vi "Process.vi"(8 "error in":errorcluster, 11 "Edit.Path":refnum<class "Edit.Path.lvclass">) -> (0 "error out":errorcluster, 3 "Edit.Path out":refnum<class "Edit.Path.lvclass">)   [LabVIEW 2019, in "Edit.Path.lvclass"]
doc: "---------------------------------------------------------------\nJKI State Machine Objects™\nhttp://jki.net/state-machine-objects/\nCopyright (C) 2005-2015, JKI <info@jki.net>\nALL RIGHTS RESERVED"
uses:
  Edit.Path.lvclass
  C:/Program Files (x86)/National Instruments/LabVIEW 2019/vi.lib/JKI/JKI SMO/SMO/SMO.lvclass
  <vilib>/JKI/JKI SMO/SMO/Typedefs/Parent Call--Enum.ctl
  Settings/ObjectSettings/ObjectSettings.lvclass/ObjectSettings.ctl
  Settings/Path Settings/Path Settings.lvclass/Path Settings.ctl
  subVIs/typedefs/Schedule Types/Schedule--Constant.ctl
  Settings/Setting Database/Setting Database.lvclass
  Settings/Path Settings/Path Settings.lvclass
  C:/Users/Albro/Documents/GitHub/AFM-Lithography/lvsrc/Classes/Settings/ObjectSettings/ObjectSettings.lvclass
  <vilib>/JKI/JKI SMO/SMO/SMO.lvclass/SMO.ctl
  <vilib>/Utility/miscctls.llb/LVPointTypeDef.ctl
  Settings/Setting Database/Typedefs/PrivateEvents--Setting Database.Copy Settings To Group.ctl
  Settings/Setting Database/Typedefs/PrivateEvents--Setting Database.SetDefaultPath.ctl
  Settings/Setting Database/Typedefs/PrivateEvents--Setting Database.CopyActivePathToAll.ctl
  Settings/ObjectSettings/Accessors/Write Voltage Schedule.vi
  Settings/ObjectSettings/Accessors/Write Speed Schedule.vi
  Settings/ObjectSettings/Accessors/Write Direction.vi
  Settings/ObjectSettings/Accessors/Write Resistance.vi
  Settings/ObjectSettings/Accessors/Write Enabled.vi
  Settings/Path Settings/Accessors/Write Fill Orientation.vi
  Settings/Path Settings/Accessors/Write Smooth Segments.vi
  Settings/ObjectSettings/Accessors/Read Speed Settings.vi
  Settings/ObjectSettings/Accessors/Read Voltage Settings.vi
  Settings/Path Settings/Accessors/Write Fill Spacing.vi
  Settings/Path Settings/Accessors/Write Interpolation.vi
  Settings/Path Settings/Accessors/Read Interpolation.vi
  Settings/ObjectSettings/Accessors/Read Enabled.vi
  Settings/ObjectSettings/Accessors/Read Direction.vi
  Settings/Path Settings/Accessors/Read Fill Orientation.vi
  Settings/Path Settings/Accessors/Read Smooth Segments.vi
  Settings/Path Settings/Accessors/Read Fill Spacing.vi
  Settings/ObjectSettings/Accessors/Read Speed Schedule.vi
  Settings/ObjectSettings/Accessors/Read Voltage Schedule.vi
  Settings/ObjectSettings/Accessors/Read Resistance.vi
  <vilib>/JKI/JKI SMO/SMO/Private/ReftoDVR--SMO.vi
  Edit/Edit.lvclass
  <vilib>/JKI/JKI SMO/SMO/SMO.lvclass
  Settings/ObjectSettings/ObjectSettings.lvclass
panel:
  in  "Apply":bool
  out "Group String":string
  out "ID String":string
  in  "Apply All":bool
  in  "Interpolation":dbl caption="Numeric 2"
  in  "Fill Spacing":dbl caption="Numeric 2"
  in  "Voltage (V)":dbl caption="Numeric 2"
  in  "Speed (um/s)":dbl caption="Numeric 2"
  in  "Smooth Segments":dbl caption="Numeric 2"
  in  "Fill Orientation":u16(ring) caption="Ring" items=["Horizontal", "Vertical"]
  in  "Deviate?":bool=TRUE
  in  "Enabled?":bool=TRUE
  in  "Set Resistance":T1(ring) caption="Enum"
  in  "Direction":u16(ring) caption="Ring" items=["Forward", "Backward"]
  in  "Speed Schedule":u16(ring) caption="Ring" items=["Constant", "Ramp", "Fn. Generator", "Formula"]
  in  "Voltage Schedule":u16(ring) caption="Ring" items=["Constant", "Ramp", "Fn. Generator", "Formula"]
  in  "Speed Settings":bool
  in  "Deviate Settings":bool
  in  "Voltage Settings":bool
  in  "Save Default":bool
  in  "Copy to All":bool
  # "For instructions on how to use the JKI State Machine Objects, examples and video tutorials, visit:\nhttp://jki.net/state-machine-objects/\n\nJKI State Machine Objects™\nhttp://jki.net/state-machine-objects/\nCopyright (C) 2005-2015, JKI <info@jki.net>\nALL RIGHTS RESERVED"
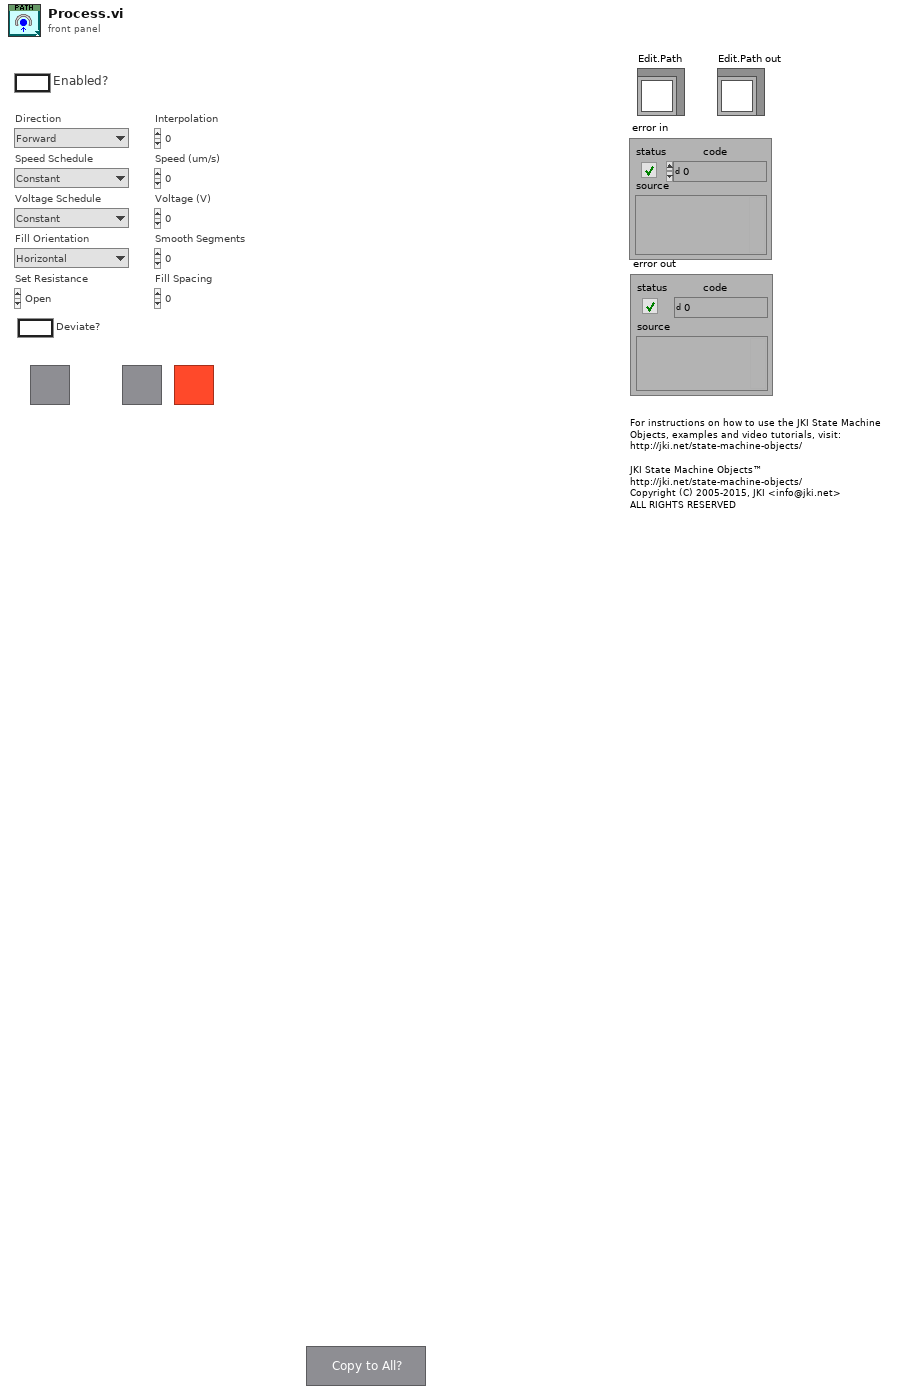
[diagram p1: front panel]
types:
  T1 = enum16{"Open", "Discharge Tip", "0 ohm", "100 kohm", "10 Mohm", "1 Gohm"}
  T2 = typedef "SMO.lvclass/Parent Call--Enum.ctl" = enum16{"Allows parent to run", "Does not request parent to run"}
  T3 = typedef "Schedule--Constant.ctl" = cluster{"Value":dbl}
  T4 = enum32{"invalid app kind", "Development System", "Run Time System", "Student Edition", "Embedded LabVIEW", "Evaluation", "Custom"}
  T5 = typedef "LVPointTypeDef.ctl" = cluster{"Horizontal":i16, "Vertical":i16}
  T6 = enum16{"Always On", "Always Off", "Off While Running"}
  T7 = enum8{"Enabled", "Disabled", "Disabled and Grayed Out"}
  T8 = enum32{"Invalid", "Standard", "Closed", "Hidden", "Minimized", "Maximized"}
  T9 = enum32{"Bad", "Idle", "Run top level", "Running"}
  T10 = typedef "Setting Database.lvclass/PrivateEvents--Setting Database.Copy Settings To Group.ctl" = cluster{"Name":string, "Group":string}
  T11 = typedef "Setting Database.lvclass/PrivateEvents--Setting Database.SetDefaultPath.ctl" = bool
  T12 = typedef "Setting Database.lvclass/PrivateEvents--Setting Database.CopyActivePathToAll.ctl" = bool
  T13 = typedef "Setting Database.lvclass/PublicEvents--Setting Database.NewActivePath.ctl" = refnum<class "Path Settings.lvclass">
  T14 = cluster{"Core":cluster{"Current VI Reference":refnum<vi>, "Close Panel on Exit?":bool, "error":errorcluster}, "Self":refnum<class "Edit.Path.lvclass">, "SettingDB":refnum<class "Setting Database.lvclass">, "Path Settings":refnum<class "Path Settings.lvclass">}
  T15 = cluster{"Current VI Reference":refnum<vi>, "Close Panel on Exit?":bool, "error":errorcluster}
  T16 = typedef "SMO.lvclass/Protected Events.ctl" = cluster{"StopProcesses":refnum<user-event>, "AbortProcesses":refnum<user-event>, "Config Changed":refnum<user-event>, "Dependency":refnum<user-event>}
  T17 = typedef "Setting Database.lvclass/PublicEvents--Cluster.ctl" = cluster{"NewActivePath":refnum<user-event>, "PathsUpdated":refnum<user-event>, "RectanglesUpdated":refnum<user-event>, "NewActiveRectangle":refnum<user-event>, "NewActiveFunnel":refnum<user-event>, "FunnelsUpdated":refnum<user-event>, "NewActiveDot":refnum<user-event>, "DotsUpdated":refnum<user-event>}
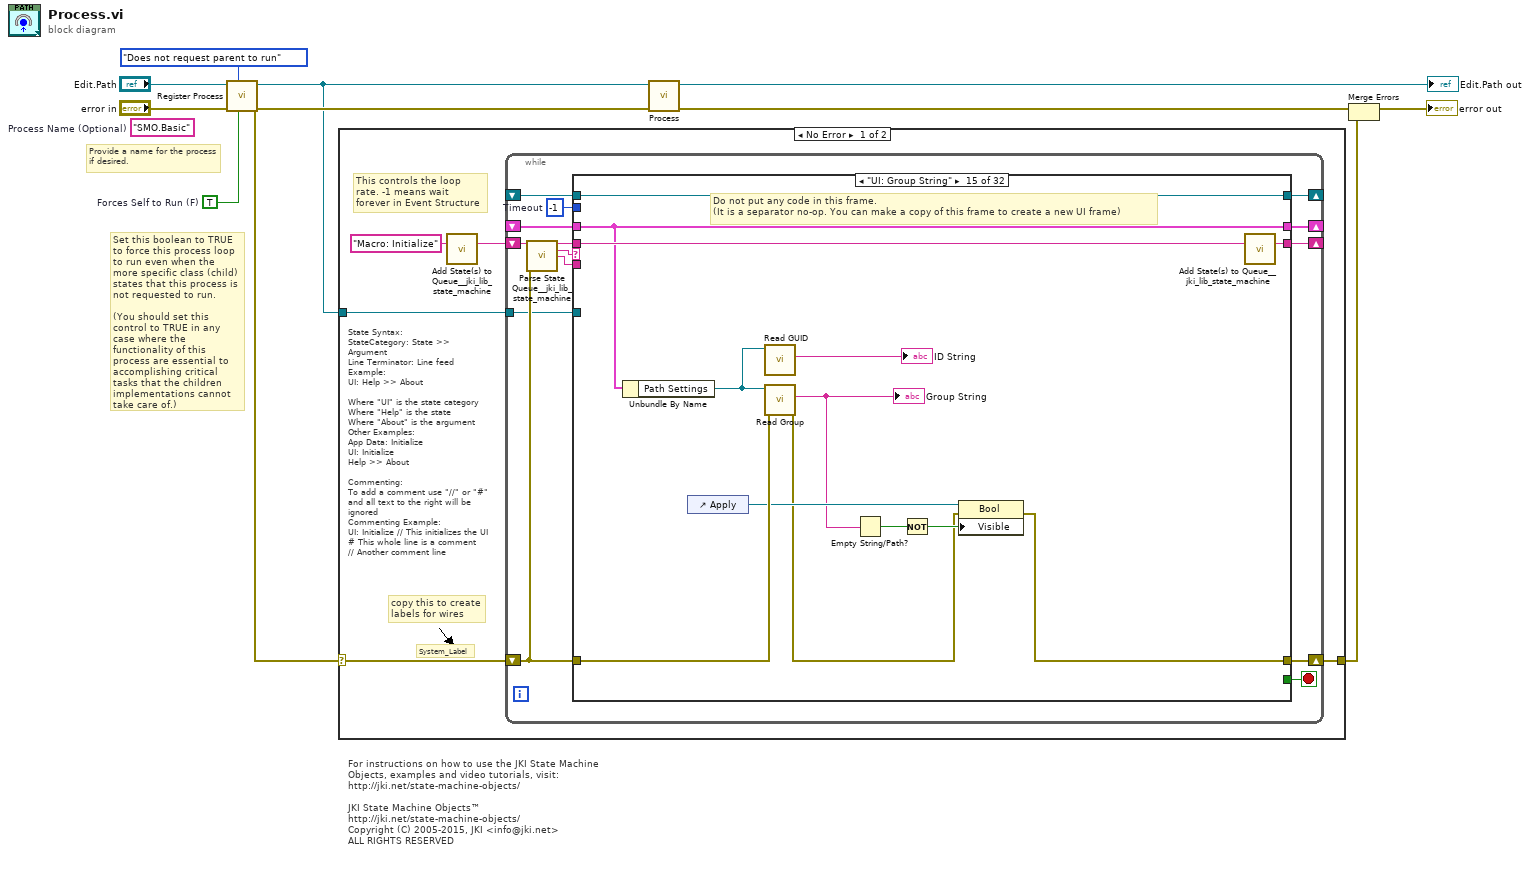
[diagram p0: block diagram]
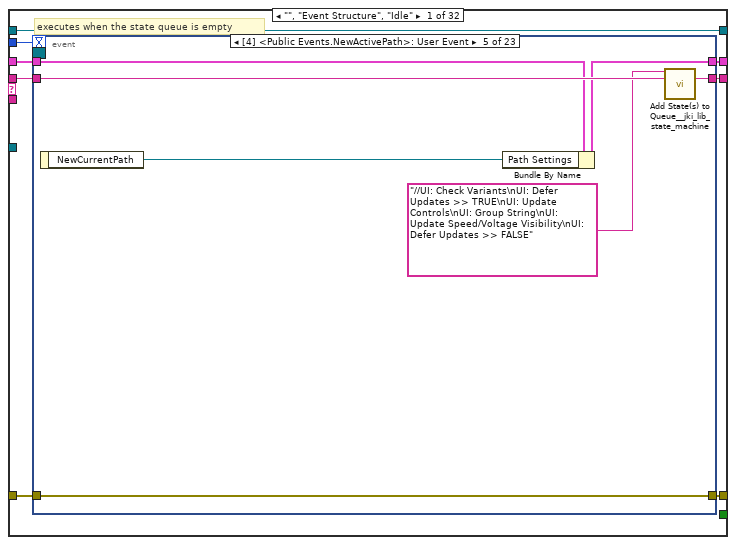
[diagram p2: hidden frame]
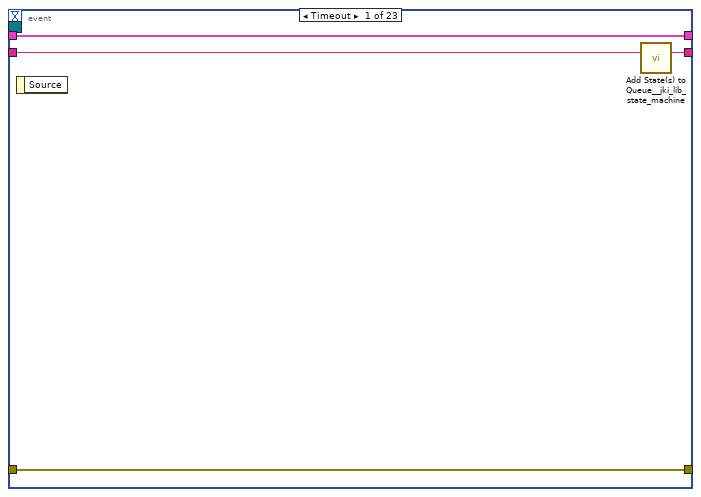
[diagram p3: hidden frame]
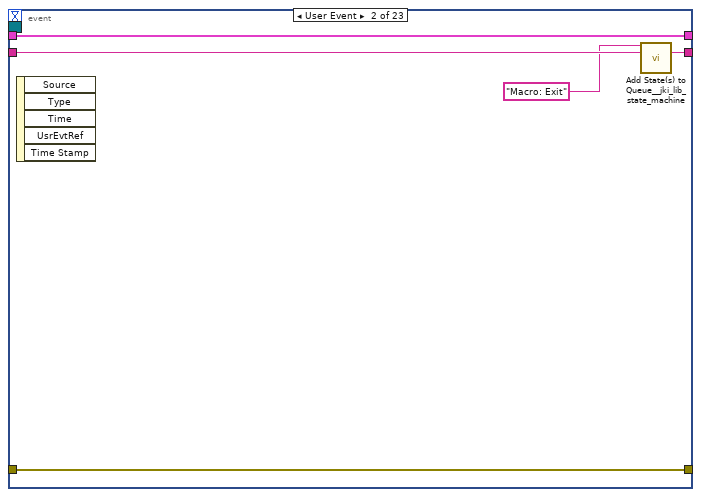
[diagram p4: hidden frame]
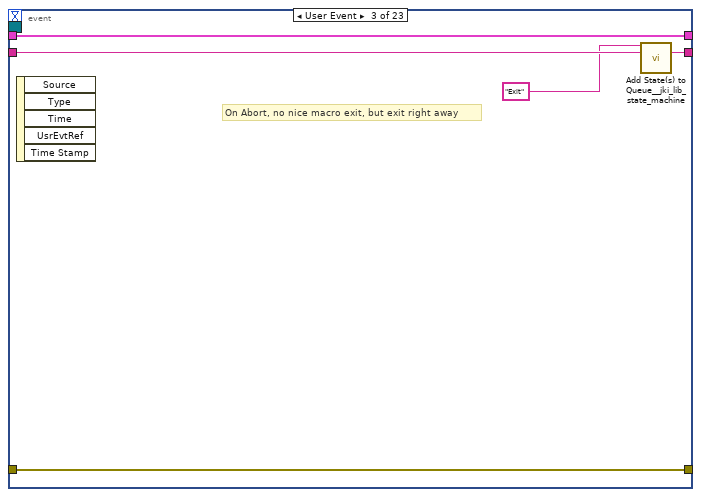
[diagram p5: hidden frame]
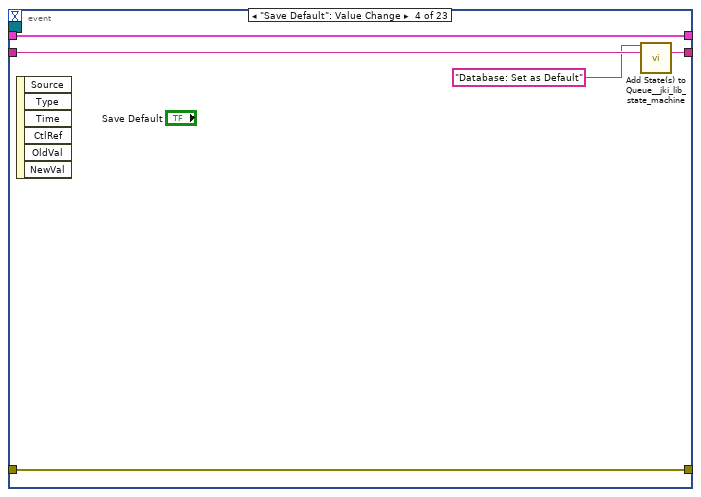
[diagram p6: hidden frame]
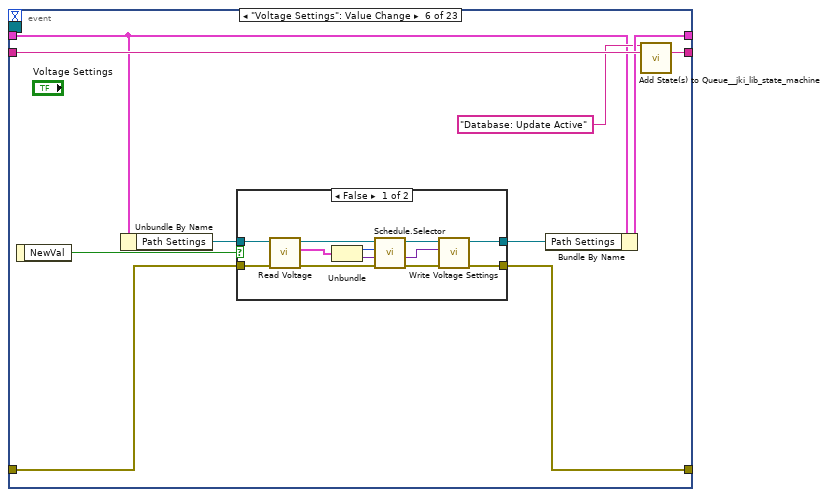
[diagram p7: hidden frame]
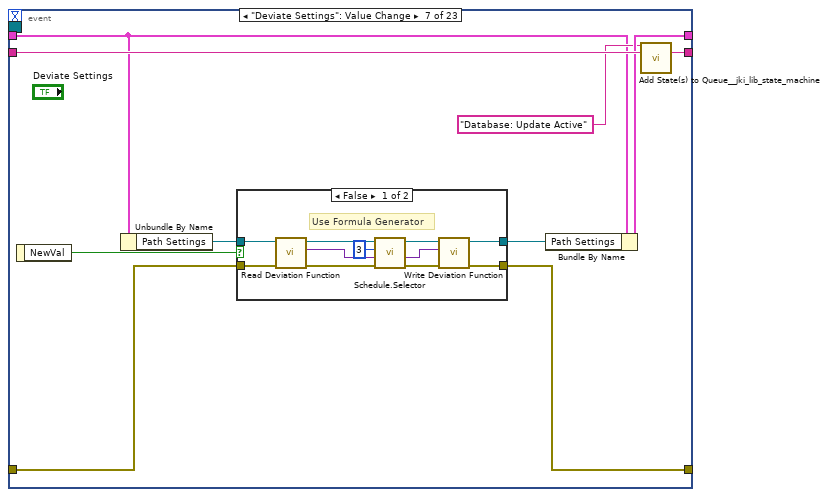
[diagram p9: hidden frame]
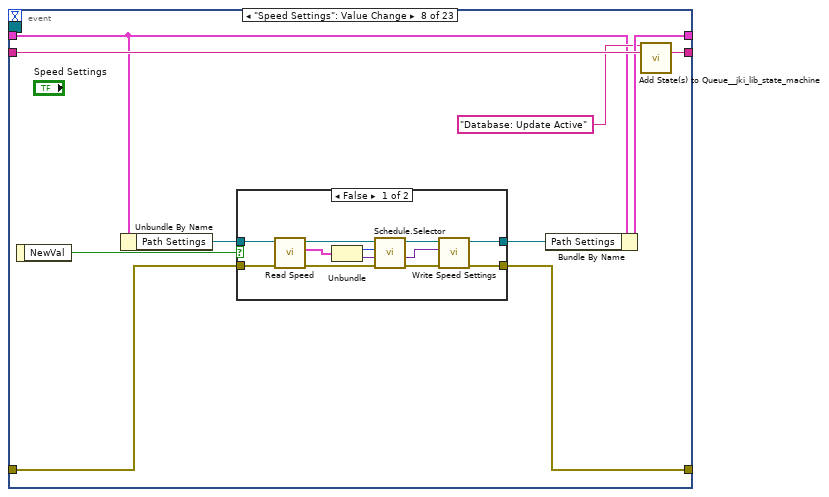
[diagram p11: hidden frame]
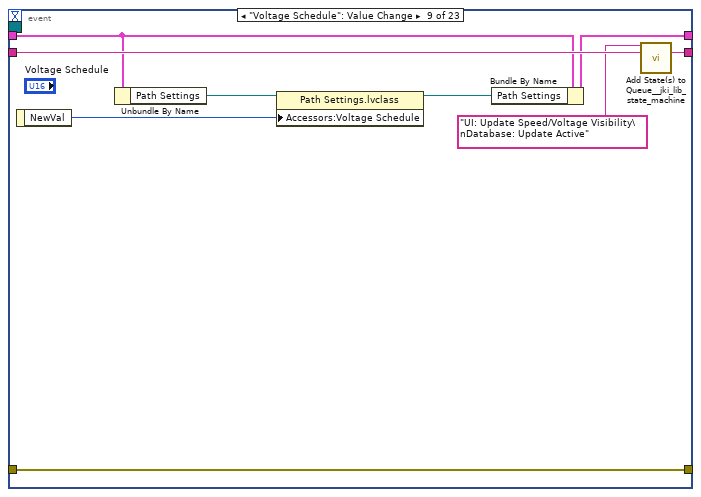
[diagram p13: hidden frame]
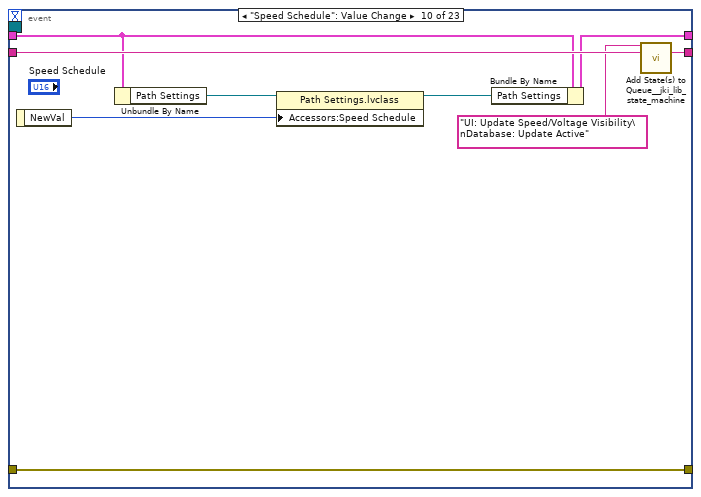
[diagram p14: hidden frame]
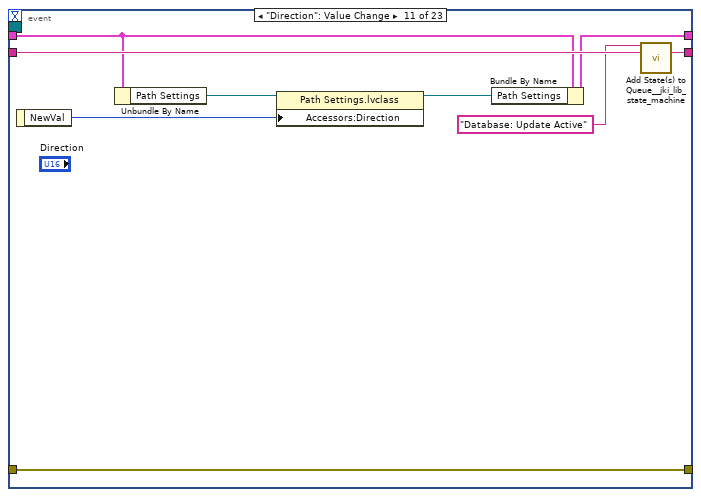
[diagram p15: hidden frame]
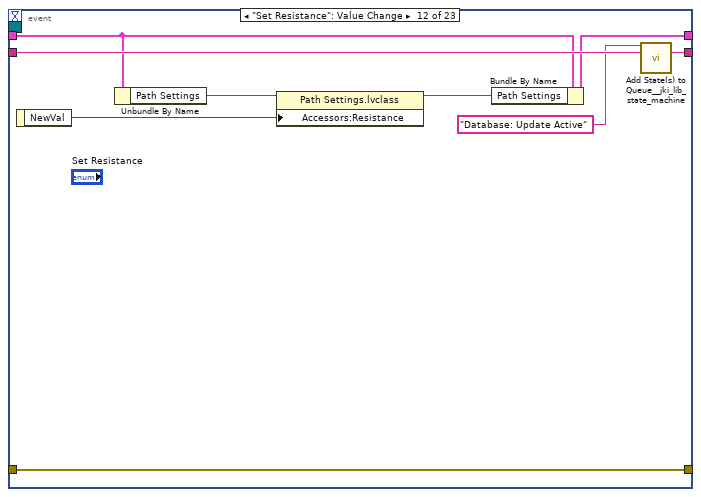
[diagram p16: hidden frame]
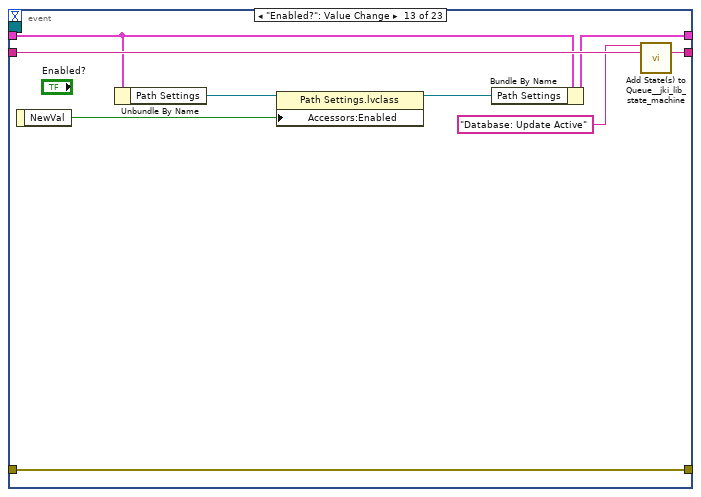
[diagram p17: hidden frame]
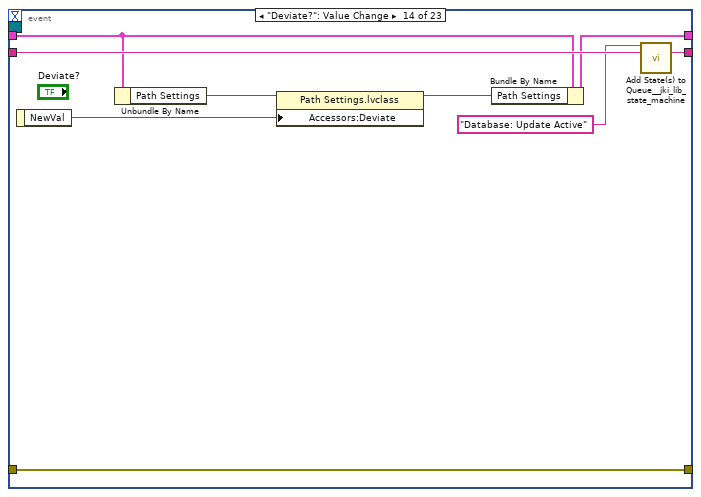
[diagram p18: hidden frame]
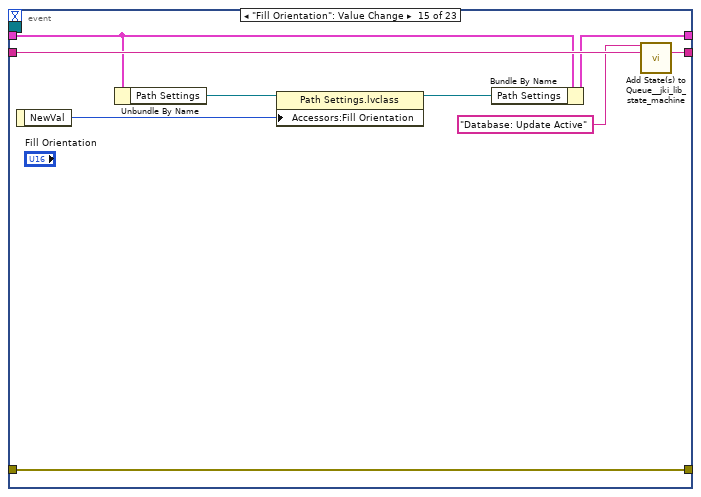
[diagram p19: hidden frame]
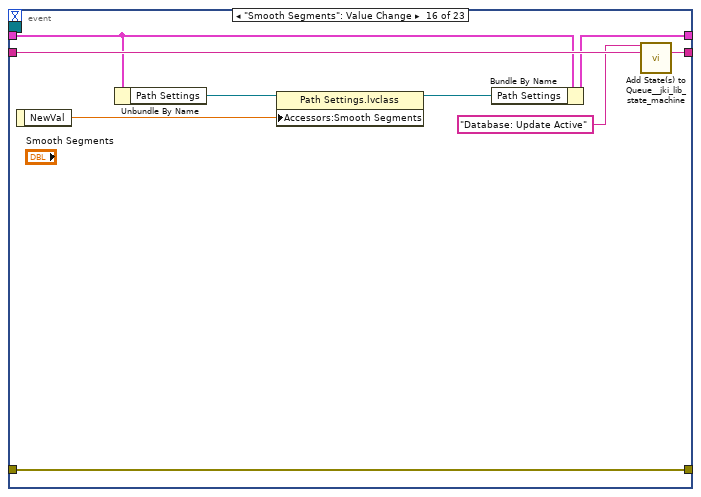
[diagram p20: hidden frame]
diagram:
  w2 = TRUE  # Forces Self to Run (F)
  (unwired) "SMO.Basic"  # Process Name (Optional)
  # "Provide a name for the process\nif desired."
  # "Set this boolean to TRUE to force this process loop to run even when the more specific class (child) states that this process is not requested to run.\n\n(You should set this control to TRUE in any case where the functionality of this process are essential to accomplishing critical tasks that the children implementations cannot take care of.)"
  # "For instructions on how to use the JKI State Machine Objects, examples and video tutorials, visit:\nhttp://jki.net/state-machine-objects/\n\nJKI State Machine Objects™\nhttp://jki.net/state-machine-objects/\nCopyright (C) 2005-2015, JKI <info@jki.net>\nALL RIGHTS RESERVED"
  n1 = call <vilib>:"Register Process.vi"("Forces Self to Run (F)"=w2, "Parent Call"=Parent_Call--Enum."Does not request parent to run", "error in (no error)"="error in", "SMO"="Edit.Path") -> ("error out"=w7:errorcluster, "SMO out"=w1:refnum<class "Edit.Path.lvclass">)  [unwired: 6 in]
  n2 = case shown="No Error" w7 {
    selector: w7 -> [w14 w651]
    tunnel: w1 -> [w13 _]
    tunnel: [w11 w651] -> w4
    frame No Error {
      # "State Syntax:\nStateCategory: State >> Argument\nLine Terminator: Line feed\nExample:\nUI: Help >> About\n\nWhere \"UI\" is the state category\nWhere \"Help\" is the state\nWhere \"About\" is the argument\nOther Examples:\nApp Data: Initialize\nUI: Initialize\nHelp >> About\n\nCommenting:\nTo add a comment use \"//\" or \"#\" and all text to the right will be ignored\nCommenting Example:\nUI: Initialize // This initializes the UI\n# This whole line is a comment\n// Another comment line"
      # "copy this to create labels for wires"
      # "This controls the loop rate. -1 means wait forever in Event Structure"
      # "System_Label"
      n3 = call <vilib>:"Add State(s) to Queue__jki_lib_state_machine.vi"("State(s) in (\"\")"="Macro: Initialize") -> ("States Out"=w12:string)  [unwired: 14 in]
      n4 = while "JKI - String-Based Queued State Machine (Basic) v1.0" {
        shift-right: [w22] -> _
        shift-left: _ -> [w20]
        shift-right: [w25] -> w11
        shift-left: w14 -> [w19]
        shift-right: [w24] -> _
        shift-left: w12 -> [w26]
        shift-right: [w18] -> _
        shift-left: _ -> [w17]
        tunnel: w13 -> [w16]
        stop <- w23 stop-if-true
        w21 = -1  # Timeout
        n5 = call <vilib>:"Parse State Queue__jki_lib_state_machine.vi"("State Queue"=w26, "Error In (no error)"=w19) -> ("Remaining States"=w28:string, "Current State"=w29:string, "Arguments"=w27:string)  [unwired: 11 in]
        n6 = case shown="\"UI: Group String\"" w29 {
          selector: w29 -> [_ _ w281 _ _ _ _ _ _ _ _ _ _ _ _ _ _ _ _ _ _ _ _ _ _ _ _ _ _ _ _ _]
          tunnel: w28 -> [w37 w275 w277 w300 w314 w320 w325 w337 w344 w349 w362 w368 w373 w384 w397 w410 w432 w459 w466 w485 w497 w529 w540 w545 w559 w573 w578 w592 w602 w619 w640 w650]
          tunnel: w27 -> [_ _ _ _ _ _ _ _ _ _ _ _ _ w375 _ _ _ _ w462 _ w493 _ _ _ _ _ _ _ _ _ _ _]
          tunnel: [w34 w273 w284 w298 errorcluster {"status"=FALSE, "code"=0, "source"=""} ("error out") w315 w323 w327 w339 w347 w355 w363 w371 w382 w387 w408 w413 w457 w463 w473 w491 w527 w532 w543 w557 w571 w576 w580 w595 w608 w632 w642] -> w25
          tunnel: w19 -> [w33 w273 w283 w298 w301 _ w323 w326 w340 w347 w353 w364 w371 w382 w393 w408 w416 w457 w464 w481 w492 w527 w531 w543 w557 w571 w576 w579 w594 w605 w631 w641]
          tunnel: [w36 w274 w282 w299 w313 w319 w324 w336 w343 w348 w361 w367 w372 w383 w396 w409 w431 w458 w465 w484 w496 w528 w539 w544 w558 w572 w577 w591 w601 w618 w639 w649] -> w24
          tunnel: [_ _ _ _ _ TRUE _ _ _ _ _ _ _ _ _ _ _ _ _ _ _ _ _ _ _ _ _ _ _ _ _ _] -> w23
          tunnel: [w32 w272 w280 w291 w303 w316 w322 w334 w341 w346 w359 w366 w370 w380 w394 w406 w423 w453 w461 w483 w490 w526 w533 w542 w556 w570 w575 w588 w599 w616 w637 w647] -> w22
          tunnel: w21 -> [w31 _ _ _ _ _ _ _ _ _ _ _ _ _ _ _ _ _ _ _ _ _ _ _ _ _ _ _ _ _ _ _]
          tunnel: w20 -> [w35 w272 w280 w292 w302 w316 w322 _ w341 w346 w359 w366 w370 w380 w394 w405 w423 w453 w461 w483 w490 w526 w533 w542 w556 w570 w575 w587 w598 w604 w636 w646]
          tunnel: [w30 w271 w276 w288 w311 w317 w321 w332 w338 w345 w360 w365 w369 w381 w395 w407 w430 w454 w460 w471 w495 w525 w538 w541 w555 w569 w574 w590 w600 w614 w638 w648] -> w18
          tunnel: w17 -> [w30 w271 w276 w288 w311 w317 w321 w332 w338 w345 _ w365 w369 w381 w395 w407 w430 w454 w460 w471 w495 w525 w538 w541 w555 w569 w574 w590 w600 w614 w638 w648]
          tunnel: w16 -> [_ _ _ _ _ _ _ w330 _ _ _ _ _ _ _ _ _ _ _ _ _ _ _ _ _ _ _ _ _ _ _ _]
          frame "", "Event Structure", "Idle" {
            # "executes when the state queue is empty"
            n7 = event shown="[4] <Public Events.NewActivePath>: User Event" {
              selector: w30 -> [_ _ _ _ _ _ _ _ _ _ _ _ _ _ _ _ _ _ _ _ _ _ _]
              dyn-events: _ -> [_ _ _ _ _ _ _ _ _ _ _ _ _ _ _ _ _ _ _ _ _ _ _]
              timeout: w31 -> [_ _ _ _ _ _ _ _ _ _ _ _ _ _ _ _ _ _ _ _ _ _ _]
              tunnel: w37 -> [w41 w46 w51 w56 w63 w73 w97 w120 w143 w152 w161 w170 w179 w188 w197 w206 w221 w236 w245 w254 w259 w264 w270]
              tunnel: [w40 w45 w50 w55 w62 w72 w96 w119 w142 w151 w160 w169 w178 w187 w196 w205 w220 w235 w244 w253 w258 w263 w269] -> w36
              tunnel: w35 -> [w38 w43 w48 w53 w59 w69 w93 w116 w136 w145 w154 w163 w172 w181 w190 w199 w216 w231 w238 w247 w257 w262 w267]
              tunnel: [w39 w44 w49 w54 w61 w65 w89 w112 w141 w150 w159 w168 w177 w186 w195 w204 w208 w223 w243 w252 w256 w261 w268] -> w34
              tunnel: w33 -> [w39 w44 w49 w54 w61 w64 w88 w111 w141 w150 w159 w168 w177 w186 w195 w204 w207 w222 w243 w252 w256 w261 w268]
              tunnel: [w38 w43 w48 w53 w60 w71 w95 w118 w140 w149 w158 w167 w176 w185 w194 w203 w219 w234 w242 w251 w257 w262 w267] -> w32
              event Timeout {
                n8 = event-data() -> ()  [unwired: 1 in, 1 out]
                n9 = call <vilib>:"Add State(s) to Queue__jki_lib_state_machine.vi"("State(s) in (\"\")"=w41) -> ("States Out"=w40:string)  [unwired: 14 in]
              }
              event User Event {
                n10 = event-data() -> ()  [unwired: 1 in, 5 out]
                n11 = call <vilib>:"Add State(s) to Queue__jki_lib_state_machine.vi"("State(s) in Front (\"\")"="Macro: Exit", "State(s) in (\"\")"=w46) -> ("States Out"=w45:string)  [unwired: 13 in]
              }
              event User Event {
                # "On Abort, no nice macro exit, but exit right away"
                n12 = event-data() -> ()  [unwired: 1 in, 5 out]
                n13 = call <vilib>:"Add State(s) to Queue__jki_lib_state_machine.vi"("State(s) in Front (\"\")"="Exit", "State(s) in (\"\")"=w51) -> ("States Out"=w50:string)  [unwired: 13 in]
              }
              event "Save Default": Value Change {
                n14 = event-data() -> ()  [unwired: 1 in, 6 out]
                n15 = call <vilib>:"Add State(s) to Queue__jki_lib_state_machine.vi"("State(s) in Front (\"\")"="Database: Set as Default", "State(s) in (\"\")"=w56) -> ("States Out"=w55:string)  [unwired: 13 in]
              }
              event User Event {
                n16 = event-data() -> ("NewCurrentPath"=w57:T13)  [unwired: 1 in]
                n17 = Bundle By Name(cluster=w59, "Path Settings"=w57) -> (w60:T14)
                n18 = call <vilib>:"Add State(s) to Queue__jki_lib_state_machine.vi"("State(s) in Front (\"\")"="//UI: Check Variants\nUI: Defer Updates >> TRUE\nUI: Update Controls\nUI: Group String\nUI: Update Speed/Voltage Visibility\nUI: Defer Updates >> FALSE", "State(s) in (\"\")"=w63) -> ("States Out"=w62:string)  [unwired: 13 in]
              }
              event "Voltage Settings": Value Change {
                n19 = event-data() -> ("NewVal"=w68:bool)  [unwired: 1 in]
                n20 = Unbundle By Name(w69) -> ("Path Settings"=w67:refnum<class "Path Settings.lvclass">)
                n21 = case shown="False" w68 {
                  tunnel: w67 -> [w85 w87]
                  tunnel: [w77 w87] -> w66
                  tunnel: w64 -> [w84 w86]
                  tunnel: [w74 w86] -> w65
                  frame False {
                    n22 = call "Read Voltage.vi"("error in (no error)"=w84, "ObjectSettings in"=w85) -> ("error out"=w82:errorcluster, "Voltage"=w81:cluster{"Schedule":u16, "Settings":variant}, "ObjectSettings out"=w83:refnum<class "Path Settings.lvclass">)  [unwired: 7 in]
                    n23 = Unbundle(w81) -> ("Schedule"=w80:u16, "Settings"=w79:variant)
                    n24 = call-dynamic "Schedule.Selector.vi"("error in (no error)"=w82, "Settings In"=w79, "Schedule"=w80, "ObjectSettings in"=w83) -> ("error out"=w76:errorcluster, "Settings Out"=w75:variant, "ObjectSettings out"=w78:refnum<class "Path Settings.lvclass">)  [unwired: 5 in]
                    n25 = call "Write Voltage Settings.vi"("error in (no error)"=w76, "Settings"=w75, "ObjectSettings in"=w78) -> ("error out"=w74:errorcluster, "ObjectSettings out"=w77:refnum<class "Path Settings.lvclass">)  [unwired: 7 in]
                  }
                  frame True {
                  }
                }
                n26 = Bundle By Name(cluster=w69, "Path Settings"=w66) -> (w71:T14)
                n27 = call <vilib>:"Add State(s) to Queue__jki_lib_state_machine.vi"("State(s) in Front (\"\")"="Database: Update Active", "State(s) in (\"\")"=w73) -> ("States Out"=w72:string)  [unwired: 13 in]
              }
              event "Deviate Settings": Value Change {
                n28 = event-data() -> ("NewVal"=w92:bool)  [unwired: 1 in]
                n29 = Unbundle By Name(w93) -> ("Path Settings"=w91:refnum<class "Path Settings.lvclass">)
                n30 = case shown="False" w92 {
                  tunnel: w91 -> [w103 w110]
                  tunnel: [w107 w110] -> w90
                  tunnel: w88 -> [w100 w109]
                  tunnel: [w104 w109] -> w89
                  frame False {
                    # "Use Formula Generator"
                    n31 = call-dynamic "Read Deviation Function.vi"("error in (no error)"=w100, "Path Settings in"=w103) -> ("error out"=w101:errorcluster, "Deviation Function"=w99:variant, "Path Settings out"=w102:refnum<class "Path Settings.lvclass">)  [unwired: 7 in]
                    n32 = call-dynamic "Schedule.Selector.vi"("error in (no error)"=w101, "Settings In"=w99, "Schedule"=u16 3, "ObjectSettings in"=w102) -> ("error out"=w106:errorcluster, "Settings Out"=w105:variant, "ObjectSettings out"=w108:refnum<class "Path Settings.lvclass">)  [unwired: 5 in]
                    n33 = call-dynamic "Write Deviation Function.vi"("error in (no error)"=w106, "Deviation Function"=w105, "Path Settings in"=w108) -> ("error out"=w104:errorcluster, "Path Settings out"=w107:refnum<class "Path Settings.lvclass">)  [unwired: 7 in]
                  }
                  frame True {
                  }
                }
                n34 = Bundle By Name(cluster=w93, "Path Settings"=w90) -> (w95:T14)
                n35 = call <vilib>:"Add State(s) to Queue__jki_lib_state_machine.vi"("State(s) in Front (\"\")"="Database: Update Active", "State(s) in (\"\")"=w97) -> ("States Out"=w96:string)  [unwired: 13 in]
              }
              event "Speed Settings": Value Change {
                n36 = event-data() -> ("NewVal"=w115:bool)  [unwired: 1 in]
                n37 = Unbundle By Name(w116) -> ("Path Settings"=w114:refnum<class "Path Settings.lvclass">)
                n38 = case shown="False" w115 {
                  tunnel: w114 -> [w130 w134]
                  tunnel: [w124 w134] -> w113
                  tunnel: w111 -> [w128 w133]
                  tunnel: [w123 w133] -> w112
                  frame False {
                    n39 = call "Read Speed.vi"("error in (no error)"=w128, "ObjectSettings in"=w130) -> ("error out"=w127:errorcluster, "Speed"=w126:cluster{"Schedule":u16, "Settings":variant}, "ObjectSettings out"=w129:refnum<class "Path Settings.lvclass">)  [unwired: 7 in]
                    n40 = Unbundle(w126) -> ("Schedule"=w132:u16, "Settings"=w131:variant)
                    n41 = call-dynamic "Schedule.Selector.vi"("error in (no error)"=w127, "Settings In"=w131, "Schedule"=w132, "ObjectSettings in"=w129) -> ("error out"=w122:errorcluster, "Settings Out"=w121:variant, "ObjectSettings out"=w125:refnum<class "Path Settings.lvclass">)  [unwired: 5 in]
                    n42 = call "Write Speed Settings.vi"("error in (no error)"=w122, "Settings"=w121, "ObjectSettings in"=w125) -> ("error out"=w123:errorcluster, "ObjectSettings out"=w124:refnum<class "Path Settings.lvclass">)  [unwired: 7 in]
                  }
                  frame True {
                  }
                }
                n43 = Bundle By Name(cluster=w116, "Path Settings"=w113) -> (w118:T14)
                n44 = call <vilib>:"Add State(s) to Queue__jki_lib_state_machine.vi"("State(s) in Front (\"\")"="Database: Update Active", "State(s) in (\"\")"=w120) -> ("States Out"=w119:string)  [unwired: 13 in]
              }
              event "Voltage Schedule": Value Change {
                n45 = event-data() -> ("NewVal"=w135:u16)  [unwired: 1 in]
                n46 = Unbundle By Name(w136) -> ("Path Settings"=w138:refnum<class "Path Settings.lvclass">)
                n47 = property class="Path Settings.lvclass"(reference=w138, "Accessors:Voltage Schedule"=w135) -> (reference out=w137:refnum<class "Path Settings.lvclass">)  [unwired: 1 in, 1 out]
                n48 = Bundle By Name(cluster=w136, "Path Settings"=w137) -> (w140:T14)
                n49 = call <vilib>:"Add State(s) to Queue__jki_lib_state_machine.vi"("State(s) in Front (\"\")"="UI: Update Speed/Voltage Visibility\nDatabase: Update Active", "State(s) in (\"\")"=w143) -> ("States Out"=w142:string)  [unwired: 13 in]
              }
              event "Speed Schedule": Value Change {
                n50 = event-data() -> ("NewVal"=w144:u16)  [unwired: 1 in]
                n51 = Unbundle By Name(w145) -> ("Path Settings"=w147:refnum<class "Path Settings.lvclass">)
                n52 = property class="Path Settings.lvclass"(reference=w147, "Accessors:Speed Schedule"=w144) -> (reference out=w146:refnum<class "Path Settings.lvclass">)  [unwired: 1 in, 1 out]
                n53 = Bundle By Name(cluster=w145, "Path Settings"=w146) -> (w149:T14)
                n54 = call <vilib>:"Add State(s) to Queue__jki_lib_state_machine.vi"("State(s) in Front (\"\")"="UI: Update Speed/Voltage Visibility\nDatabase: Update Active", "State(s) in (\"\")"=w152) -> ("States Out"=w151:string)  [unwired: 13 in]
              }
              event "Direction": Value Change {
                n55 = event-data() -> ("NewVal"=w153:u16)  [unwired: 1 in]
                n56 = Unbundle By Name(w154) -> ("Path Settings"=w156:refnum<class "Path Settings.lvclass">)
                n57 = property class="Path Settings.lvclass"(reference=w156, "Accessors:Direction"=w153) -> (reference out=w155:refnum<class "Path Settings.lvclass">)  [unwired: 1 in, 1 out]
                n58 = Bundle By Name(cluster=w154, "Path Settings"=w155) -> (w158:T14)
                n59 = call <vilib>:"Add State(s) to Queue__jki_lib_state_machine.vi"("State(s) in Front (\"\")"="Database: Update Active", "State(s) in (\"\")"=w161) -> ("States Out"=w160:string)  [unwired: 13 in]
              }
              event "Set Resistance": Value Change {
                n60 = event-data() -> ("NewVal"=w162:T1)  [unwired: 1 in]
                n61 = Unbundle By Name(w163) -> ("Path Settings"=w165:refnum<class "Path Settings.lvclass">)
                n62 = property class="Path Settings.lvclass"(reference=w165, "Accessors:Resistance"=w162) -> (reference out=w164:refnum<class "Path Settings.lvclass">)  [unwired: 1 in, 1 out]
                n63 = Bundle By Name(cluster=w163, "Path Settings"=w164) -> (w167:T14)
                n64 = call <vilib>:"Add State(s) to Queue__jki_lib_state_machine.vi"("State(s) in Front (\"\")"="Database: Update Active", "State(s) in (\"\")"=w170) -> ("States Out"=w169:string)  [unwired: 13 in]
              }
              event "Enabled?": Value Change {
                n65 = event-data() -> ("NewVal"=w171:bool)  [unwired: 1 in]
                n66 = Unbundle By Name(w172) -> ("Path Settings"=w174:refnum<class "Path Settings.lvclass">)
                n67 = property class="Path Settings.lvclass"(reference=w174, "Accessors:Enabled"=w171) -> (reference out=w173:refnum<class "Path Settings.lvclass">)  [unwired: 1 in, 1 out]
                n68 = Bundle By Name(cluster=w172, "Path Settings"=w173) -> (w176:T14)
                n69 = call <vilib>:"Add State(s) to Queue__jki_lib_state_machine.vi"("State(s) in Front (\"\")"="Database: Update Active", "State(s) in (\"\")"=w179) -> ("States Out"=w178:string)  [unwired: 13 in]
              }
              event "Deviate?": Value Change {
                n70 = event-data() -> ("NewVal"=w180:bool)  [unwired: 1 in]
                n71 = Unbundle By Name(w181) -> ("Path Settings"=w183:refnum<class "Path Settings.lvclass">)
                n72 = property class="Path Settings.lvclass"(reference=w183, "Accessors:Deviate"=w180) -> (reference out=w182:refnum<class "Path Settings.lvclass">)  [unwired: 1 in, 1 out]
                n73 = Bundle By Name(cluster=w181, "Path Settings"=w182) -> (w185:T14)
                n74 = call <vilib>:"Add State(s) to Queue__jki_lib_state_machine.vi"("State(s) in Front (\"\")"="Database: Update Active", "State(s) in (\"\")"=w188) -> ("States Out"=w187:string)  [unwired: 13 in]
              }
              event "Fill Orientation": Value Change {
                n75 = event-data() -> ("NewVal"=w189:u16)  [unwired: 1 in]
                n76 = Unbundle By Name(w190) -> ("Path Settings"=w192:refnum<class "Path Settings.lvclass">)
                n77 = property class="Path Settings.lvclass"(reference=w192, "Accessors:Fill Orientation"=w189) -> (reference out=w191:refnum<class "Path Settings.lvclass">)  [unwired: 1 in, 1 out]
                n78 = Bundle By Name(cluster=w190, "Path Settings"=w191) -> (w194:T14)
                n79 = call <vilib>:"Add State(s) to Queue__jki_lib_state_machine.vi"("State(s) in Front (\"\")"="Database: Update Active", "State(s) in (\"\")"=w197) -> ("States Out"=w196:string)  [unwired: 13 in]
              }
              event "Smooth Segments": Value Change {
                n80 = event-data() -> ("NewVal"=w198:dbl)  [unwired: 1 in]
                n81 = Unbundle By Name(w199) -> ("Path Settings"=w201:refnum<class "Path Settings.lvclass">)
                n82 = property class="Path Settings.lvclass"(reference=w201, "Accessors:Smooth Segments"=w198) -> (reference out=w200:refnum<class "Path Settings.lvclass">)  [unwired: 1 in, 1 out]
                n83 = Bundle By Name(cluster=w199, "Path Settings"=w200) -> (w203:T14)
                n84 = call <vilib>:"Add State(s) to Queue__jki_lib_state_machine.vi"("State(s) in Front (\"\")"="Database: Update Active", "State(s) in (\"\")"=w206) -> ("States Out"=w205:string)  [unwired: 13 in]
              }
              event "Speed (um/s)": Value Change {
                n85 = event-data() -> ("NewVal"=w214:dbl)  [unwired: 1 in]
                n86 = Unbundle By Name(w216) -> ("Path Settings"=w213:refnum<class "Path Settings.lvclass">)
                n87 = property class="Path Settings.lvclass"(reference=w213) -> (reference out=w212:refnum<class "Path Settings.lvclass">, "Accessors:Speed Settings"=w211:variant)  [unwired: 1 in, 1 out]
                n88 = Bundle By Name(cluster=T3 {"Value"=10.0} ("Constant"), "Value"=w214) -> (w209:T3)
                n89 = call "Schedule.Write.vi"("error in (no error)"=w207, "Data to Write"=w209, "LUT In"=w211) -> ("error out"=w208:errorcluster, "LUT Out"=w210:variant)  [unwired: 7 in]
                n90 = property class="Path Settings.lvclass"(reference=w212, "Accessors:Speed Settings"=w210) -> (reference out=w217:refnum<class "Path Settings.lvclass">)  [unwired: 1 in, 1 out]
                n91 = Bundle By Name(cluster=w216, "Path Settings"=w217) -> (w219:T14)
                n92 = call <vilib>:"Add State(s) to Queue__jki_lib_state_machine.vi"("State(s) in Front (\"\")"="Database: Update Active", "State(s) in (\"\")"=w221) -> ("States Out"=w220:string)  [unwired: 13 in]
              }
              event "Voltage (V)": Value Change {
                n93 = event-data() -> ("NewVal"=w229:dbl)  [unwired: 1 in]
                n94 = Unbundle By Name(w231) -> ("Path Settings"=w228:refnum<class "Path Settings.lvclass">)
                n95 = property class="Path Settings.lvclass"(reference=w228) -> (reference out=w227:refnum<class "Path Settings.lvclass">, "Accessors:Voltage Settings"=w226:variant)  [unwired: 1 in, 1 out]
                n96 = Bundle By Name(cluster=T3 {"Value"=10.0} ("Constant"), "Value"=w229) -> (w224:T3)
                n97 = call "Schedule.Write.vi"("error in (no error)"=w222, "Data to Write"=w224, "LUT In"=w226) -> ("error out"=w223:errorcluster, "LUT Out"=w225:variant)  [unwired: 7 in]
                n98 = property class="Path Settings.lvclass"(reference=w227, "Accessors:Voltage Settings"=w225) -> (reference out=w232:refnum<class "Path Settings.lvclass">)  [unwired: 1 in, 1 out]
                n99 = Bundle By Name(cluster=w231, "Path Settings"=w232) -> (w234:T14)
                n100 = call <vilib>:"Add State(s) to Queue__jki_lib_state_machine.vi"("State(s) in Front (\"\")"="Database: Update Active", "State(s) in (\"\")"=w236) -> ("States Out"=w235:string)  [unwired: 13 in]
              }
              event "Fill Spacing": Value Change {
                n101 = event-data() -> ("NewVal"=w237:dbl)  [unwired: 1 in]
                n102 = Unbundle By Name(w238) -> ("Path Settings"=w240:refnum<class "Path Settings.lvclass">)
                n103 = property class="Path Settings.lvclass"(reference=w240, "Accessors:Fill Spacing"=w237) -> (reference out=w239:refnum<class "Path Settings.lvclass">)  [unwired: 1 in, 1 out]
                n104 = Bundle By Name(cluster=w238, "Path Settings"=w239) -> (w242:T14)
                n105 = call <vilib>:"Add State(s) to Queue__jki_lib_state_machine.vi"("State(s) in Front (\"\")"="Database: Update Active", "State(s) in (\"\")"=w245) -> ("States Out"=w244:string)  [unwired: 13 in]
              }
              event "Interpolation": Value Change {
                n106 = event-data() -> ("NewVal"=w246:dbl)  [unwired: 1 in]
                n107 = Unbundle By Name(w247) -> ("Path Settings"=w249:refnum<class "Path Settings.lvclass">)
                n108 = property class="Path Settings.lvclass"(reference=w249, "Accessors:Interpolation"=w246) -> (reference out=w248:refnum<class "Path Settings.lvclass">)  [unwired: 1 in, 1 out]
                n109 = Bundle By Name(cluster=w247, "Path Settings"=w248) -> (w251:T14)
                n110 = call <vilib>:"Add State(s) to Queue__jki_lib_state_machine.vi"("State(s) in Front (\"\")"="Database: Update Active", "State(s) in (\"\")"=w254) -> ("States Out"=w253:string)  [unwired: 13 in]
              }
              event "Copy to All", "Apply All": Value Change {
                n111 = event-data() -> ()  [unwired: 1 in, 1 out]
                n112 = call <vilib>:"Add State(s) to Queue__jki_lib_state_machine.vi"("State(s) in Front (\"\")"="Database: Copy to All", "State(s) in (\"\")"=w259) -> ("States Out"=w258:string)  [unwired: 13 in]
              }
              event "Apply": Value Change {
                n113 = event-data() -> ()  [unwired: 1 in, 1 out]
                n114 = call <vilib>:"Add State(s) to Queue__jki_lib_state_machine.vi"("State(s) in Front (\"\")"="Database: Copy to Group", "State(s) in (\"\")"=w264) -> ("States Out"=w263:string)  [unwired: 13 in]
              }
              event Panel Close? {
                # "Discard the event because we'll close the front panel ourselves in Macro: Exit"
                # "Close Panel button (pressed) Event\n(this executes Macro: Exit to terminate the VI)"
                n115 = event-data() -> ()  [unwired: 1 in, 1 out]
                n116 = event-data("Discard?"=TRUE) -> ()  [unwired: 1 in, 1 out]
                n117 = call <vilib>:"Add State(s) to Queue__jki_lib_state_machine.vi"("State(s) in Front (\"\")"="Macro: Exit", "State(s) in (\"\")"=w270) -> ("States Out"=w269:string)  [unwired: 13 in]
              }
            }
          }
          frame "---------- Core ----------" {
            # "Do not put any code in this frame.\n(it is a separator no-op)"
            n118 = call <vilib>:"Add State(s) to Queue__jki_lib_state_machine.vi"("State(s) in (\"\")"=w275) -> ("States Out"=w274:string)  [unwired: 14 in]
          }
          frame Default {
            w287 = 42 items=["No error", "Argument error", "Memory is full", "Out of zone", "End of file", "File already open", "Generic file I/O error", "File not found", "File permission error", "Disk is full", "Duplicate path", "Too many files open", "System feature not enabled", "Resource file not found", "Cannot add resource", "Resource not found", "Image not found", "Image memory error", "Pen does not exist", "Config type invalid", "Config token not found", "Config parse error", "Config memory error", "Bad external code format", "Bad external code offset", "External code not present", "Null window", "Destroy window error", "Null menu", "Print aborted", "Bad print record", "Print driver error", "Windows error during printing", "Memory error during printing", "Print dialog error", "Generic print error", "Invalid device refnum", "Device not found", "Device parameter error", "Device unit error", "Cannot open device", "Device call aborted", "Generic error", "Cancelled by user", "Object ID too low", "Object ID too high", "Object not in heap", "Unknown heap", "Unknown object (invalid DefProc)", "Unknown object (DefProc not in table)", "Message out of range", "Invalid (null) method", "Unknown message", "Manager call not supported", "Bad address", "Network operation in progress", "Network operation timed out", "Connection is busy", "Network attribute not supported", "Network error", "Address in use", "System out of memory", "Connection aborted", "Connection refused", "Not connected", "Already connected", "Connection closed", "Initialization error (interapplication manager)", "Bad occurrence", "Wait on unbound occurrence handler", "Occurrence queue overflow", "Datalog type conflict", "Unused", "Unrecognized type (interapplication manager)", "Memory corrupt", "Failed to make temporary DLL", "Old CIN version", "Drag socket not found", "Failed to load drop-object", "Failed to register OLE object", "Failed to release OLE object", "Format specifier type mismatch", "Unknown format specifier", "Too few format specifiers", "Too many format specifiers", "Scan failed", "Newer CIN version", "Error converting to variant", "Runtime menu error", "Password tampered", "Variant attribute not found", "Incompatible variant data type", "Event data is not available", "Event Store is not present", "Occurrence is not found", "Event Queue is not created", "Event info is not available", "Refnum passed is NULL", "Error retrieving Class GUID", "Error retrieving CoClass GUID", "Error retrieving TypeLib GUID.", "Bad built application magic bytes.", "Specific driver is different from the specific driver associated with the Logical Name.", "There is no session opened to the class driver.", "Max Error", "MAX - Error with config objects", "MAX - Error loading configuration", "MAX - Group not supported"]
            # "Current State"
            # "Do not delete, rename, or modify this frame.\n(this is used to capture unhandled states and typos)"
            # "Handle mistyped state name (developer tool)"
            n119 = Format Into String(format string="Software Exception: Unhandled State \"%s\"." ("message"), error in=w283, w281) -> (resulting string=w286:string, error out=w285:errorcluster)  [unwired: 1 in]
            n120 = call <vilib>:"Error Cluster From Error Code.vi"("show call chain? (False)"=TRUE, "error in (no error)"=w285, "error message (\"\")"=w286, "error code (0)"=w287) -> ("error out"=w284:errorcluster)  [unwired: 5 in]
            n121 = call <vilib>:"Add State(s) to Queue__jki_lib_state_machine.vi"("State(s) in (\"\")"=w277) -> ("States Out"=w282:string)  [unwired: 14 in]
          }
          frame "Initialize Core Data" {
            # "exe?"
            # "If panel starts closed or is an EXE, then close it when we exit"
            # "Do not delete, rename, or modify this frame.\n(this is used to determine panel behavior on exit)"
            n122 = control-ref of="Current VI Reference"() -> (w297:refnum<vi>)
            n123 = property class="VI"() -> ("Front Panel.Open"=w296:bool)  [unwired: 2 in, 2 out]
            n124 = property class="App"() -> ("App.Kind"=w295:T4)  [unwired: 2 in, 2 out]
            n125 = Not(x=w296) -> (.not. x?=w290:bool)
            n126 = Equal?(x=w295, y=T4."Run Time System" ("Application:Kind")) -> (x = y?=w289:bool)
            n127 = Or(x=w290, y=w289) -> (x .or. y?=w293:bool)
            n128 = Bundle By Name(cluster=w292, "Core.Current VI Reference"=w297, "Core.Close Panel on Exit?"=w293) -> (w291:T14)
            n129 = call <vilib>:"Add State(s) to Queue__jki_lib_state_machine.vi"("State(s) in (\"\")"=w300) -> ("States Out"=w299:string)  [unwired: 14 in]
          }
          frame "Error Handler" {
            w305 = TRUE  # Stop on Unhandled Error (T)
            # "Overwrite this method to handle errors and pass to parent if not handled. Parent will fire a public event if the error is not handled up the chain of classes."
            # "Handle any errors here.\nYou can also output any states to clean-up after errors occur"
            # "Clear error"
            n130 = Unbundle By Name(w302) -> ("Self"=w310:refnum<class "Edit.Path.lvclass">)
            n131 = call-dynamic "Handle Error.vi"("Stop on Unhandled Error (T)"=w305, "error in"=w301, "SMO"=w310) -> ("handling error"=w306:errorcluster, "Unhandled error"=w309:errorcluster)  [unwired: 6 in, 1 out]
            n132 = Bundle By Name(cluster=w302, "Core.error"=w309) -> (w303:T14)
            n133 = Select(t="Exit", s=w306, f="") -> (s? t:f=w304:string)
            n134 = call <vilib>:"Add State(s) to Queue__jki_lib_state_machine.vi"("State(s) in Front (\"\")"=w304, "State(s) in (\"\")"=w314) -> ("States Out"=w313:string)  [unwired: 13 in]
          }
          frame "Exit" {
            # "Do not put any code in this frame.\n(No errors that occur here will be handled.)"
            n135 = Unbundle By Name(w316) -> ("Core.error"=w315:errorcluster)
            n136 = call <vilib>:"Add State(s) to Queue__jki_lib_state_machine.vi"("State(s) in (\"\")"=w320) -> ("States Out"=w319:string)  [unwired: 14 in]
          }
          frame "---------- Data ----------" {
            # "Do not put any code in this frame.\n(It is a separator no-op. You can make a copy of this frame to create a new Data frame)"
            n137 = call <vilib>:"Add State(s) to Queue__jki_lib_state_machine.vi"("State(s) in (\"\")"=w325) -> ("States Out"=w324:string)  [unwired: 14 in]
          }
          frame "Data: Initialize" {
            w329 = refnum<class "Edit.Path.lvclass"> refnum  # Self
            w331 = refnum<class "Path Settings.lvclass"> refnum  # Path Settings
            w333 = refnum<class "Setting Database.lvclass"> refnum  # SettingDB
            w335 = T15 {"Current VI Reference"=refnum, "Close Panel on Exit?"=FALSE, "error"={"status"=FALSE, "code"=0, "source"=""}}  # Core
            # "Initialize the shift-register data, here.\n(data names are defined by what you wire into the bundle function)"
            n138 = Variant To Data(error in=w326, type=w329, Variant=w330) -> (data=w328:refnum<class "Edit.Path.lvclass">, error out=w327:errorcluster)
            n139 = Bundle("Core"=w335, "Self"=w328, "SettingDB"=w333, "Path Settings"=w331) -> (w334:T14)  [unwired: 1 in]
            n140 = call <vilib>:"Add State(s) to Queue__jki_lib_state_machine.vi"("State(s) in (\"\")"=w337) -> ("States Out"=w336:string)  [unwired: 14 in]
          }
          frame "Data: Cleanup" {
            # "Cleanup any data and references, here.\n(this is called automatically, by the Macro: Exit)"
            n141 = Unbundle By Name(w341) -> ("Core.Current VI Reference"=w342:refnum<vi>)
            n142 = Close Reference(reference=w342, error in (no error)=w340) -> (error out=w339:errorcluster)
            n143 = call <vilib>:"Add State(s) to Queue__jki_lib_state_machine.vi"("State(s) in (\"\")"=w344) -> ("States Out"=w343:string)  [unwired: 14 in]
          }
          frame "---------- Events ----------" {
            # "Do not put any code in this frame.\n(It is a separator no-op. You can make a copy of this frame to create a new UI frame)"
            n144 = call <vilib>:"Add State(s) to Queue__jki_lib_state_machine.vi"("State(s) in (\"\")"=w349) -> ("States Out"=w348:string)  [unwired: 14 in]
          }
          frame "Events: Register" {
            # "Do not put any code in this frame.\n(It is a separator no-op. You can make a copy of this frame to create a new UI frame)"
            n145 = Unbundle By Name(w359) -> ("Self"=w352:refnum<class "Edit.Path.lvclass">, "SettingDB"=w358:refnum<class "Setting Database.lvclass">)
            n146 = call <vilib>:"GetProtectedEvents.vi"("SMO"=w352) -> ("error out"=w350:errorcluster, "SMO Protected Events"=w351:T16)  [unwired: 8 in, 1 out]
            n147 = call "Setting Database.GetPublicEvents.vi"("Setting Database"=w358) -> ("error out"=w354:errorcluster, "Public Events"=w357:T17)  [unwired: 8 in, 1 out]
            n148 = register-events(w351, w357) -> (reference out=w360:refnum<event-registration>, error out=w356:errorcluster)  [unwired: 2 in]
            n149 = Merge Errors(w353, w356, w354, w350) -> (w355:errorcluster)
            n150 = call <vilib>:"Add State(s) to Queue__jki_lib_state_machine.vi"("State(s) in (\"\")"=w362) -> ("States Out"=w361:string)  [unwired: 14 in]
          }
          frame "Events: Unregister" {
            # "Do not put any code in this frame.\n(It is a separator no-op. You can make a copy of this frame to create a new UI frame)"
            n151 = Unregister For Events(event registration refnum=w365, error in=w364) -> (error out=w363:errorcluster)
            n152 = call <vilib>:"Add State(s) to Queue__jki_lib_state_machine.vi"("State(s) in (\"\")"=w368) -> ("States Out"=w367:string)  [unwired: 14 in]
          }
          frame "---------- UI ----------" {
            # "Do not put any code in this frame.\n(It is a separator no-op. You can make a copy of this frame to create a new UI frame)"
            n153 = call <vilib>:"Add State(s) to Queue__jki_lib_state_machine.vi"("State(s) in (\"\")"=w373) -> ("States Out"=w372:string)  [unwired: 14 in]
          }
          frame "UI: Defer Updates" {
            # "Do not put any code in this frame.\n(It is a separator no-op. You can make a copy of this frame to create a new UI frame)"
            n154 = Unbundle By Name(w380) -> ("Core.Current VI Reference"=w379:refnum<vi>)
            n155 = Match True/False String(2:"FALSE" ("false string"), 3:"TRUE" ("true string"), 4:w375) -> (0:w374:bool)  [unwired: 1 out]
            n156 = property class="VI"(reference=w379) -> ("Panel"=w378:refnum<vi>)  [unwired: 1 in, 2 out]
            n157 = property class="Pnl"(reference=w378, "DeferPanUpdts"=w374) -> ()  [unwired: 1 in, 2 out]
            n158 = call <vilib>:"Add State(s) to Queue__jki_lib_state_machine.vi"("State(s) in (\"\")"=w384) -> ("States Out"=w383:string)  [unwired: 14 in]
          }
          frame "UI: Group String" {
            # "Do not put any code in this frame.\n(It is a separator no-op. You can make a copy of this frame to create a new UI frame)"
            n159 = Unbundle By Name(w394) -> ("Path Settings"=w386:refnum<class "Path Settings.lvclass">)
            n160 = control-ref of="Apply"() -> (w392:refnum<vi>)
            n161 = call-dynamic "Read GUID.vi"("ObjectSettings in"=w386) -> ("GUID"=→"ID String":string)  [unwired: 8 in, 2 out]
            n162 = call-dynamic "Read Group.vi"("error in (no error)"=w393, "ObjectSettings in"=w386) -> ("error out"=w388:errorcluster, "Group"=w391:string)  [unwired: 7 in, 1 out]
            "Group String" <- w391
            n163 = Empty String/Path?(string/path=w391) -> (empty?=w390:bool)
            n164 = Not(x=w390) -> (.not. x?=w389:bool)
            n165 = property class="Bool"(reference=w392, error in=w388, "Visible"=w389) -> (error out=w387:errorcluster)  [unwired: 1 out]
            n166 = call <vilib>:"Add State(s) to Queue__jki_lib_state_machine.vi"("State(s) in (\"\")"=w397) -> ("States Out"=w396:string)  [unwired: 14 in]
          }
          frame "UI: Check Variants" {
            # "Do not put any code in this frame.\n(It is a separator no-op. You can make a copy of this frame to create a new UI frame)"
            n167 = Unbundle By Name(w405) -> ("Path Settings"=w404:refnum<class "Path Settings.lvclass">)
            n168 = property class="Path Settings.lvclass"(reference=w404) -> (reference out=w403:refnum<class "Path Settings.lvclass">, "Accessors:Speed Settings"=w401:variant, "Accessors:Voltage Settings"=w399:variant)  [unwired: 1 in, 1 out]
            n169 = call "Schedule.CheckVariantAttributes.vi"("Variant In"=w401) -> ("Variant Out"=w400:variant)  [unwired: 9 in, 1 out]
            n170 = call "Schedule.CheckVariantAttributes.vi"("Variant In"=w399) -> ("Variant Out"=w398:variant)  [unwired: 9 in, 1 out]
            n171 = property class="Path Settings.lvclass"(reference=w403, "Accessors:Speed Settings"=w400, "Accessors:Voltage Settings"=w398) -> (reference out=w402:refnum<class "Path Settings.lvclass">)  [unwired: 1 in, 1 out]
            n172 = Bundle By Name(cluster=w405, "Path Settings"=w402) -> (w406:T14)
            n173 = call <vilib>:"Add State(s) to Queue__jki_lib_state_machine.vi"("State(s) in (\"\")"=w410) -> ("States Out"=w409:string)  [unwired: 14 in]
          }
          frame "UI: Initialize" {
            # "Initialize the User Interface, here.\n(this is called automatically, by the Macro: Init)"
            n174 = Unbundle By Name(w423) -> ("Core.Current VI Reference"=w418:refnum<vi>)
            n175 = control-ref of="Speed Schedule"() -> (w429:refnum<vi>)
            n176 = property class="VI"(reference=w418, error in=w416) -> (error out=w415:errorcluster, "Panel"=w422:refnum<vi>)  [unwired: 1 out]
            n177 = property class="Ring (strict)"(reference=w429, error in=w416, "DisabledEnum"=T7."Disabled and Grayed Out" ("Disabled")) -> (error out=w426:errorcluster)  [unwired: 1 out]
            n178 = property class="Pnl"(reference=w422, error in=w415) -> (error out=w414:errorcluster, "Panes[]"=w421:refnum<vi>[])  [unwired: 1 out]
            n179 = Index Array(array=w421) -> (element=w420:refnum<vi>)  [unwired: 1 in]
            n180 = control-ref of="Apply All"() -> (w424:refnum<vi>)
            n181 = property class="Pane"(reference=w420, error in=w414, "HorizScrollbarVisibility"=T6."Off While Running" ("Horizontal Scrollbar Visibility"), "VertScrollbarVisibility"=T6."Off While Running" ("Horizontal Scrollbar Visibility"), "Origin"=T5 {"Horizontal"=0, "Vertical"=0}) -> (error out=w412:errorcluster)  [unwired: 1 out]
            n182 = property class="Bool"(reference=w424, error in=w426, "Colors [4]"=cluster{u32, u32}[] [{16730410, 16730410}, {16730410, 16730410}, {16730410, 16730410}, {16730410, 16730410}]) -> (error out=w425:errorcluster)  [unwired: 1 out]
            n183 = Merge Errors(w425, w412) -> (w413:errorcluster)
            n184 = call <vilib>:"Add State(s) to Queue__jki_lib_state_machine.vi"("State(s) in (\"\")"=w432) -> ("States Out"=w431:string)  [unwired: 14 in]
          }
          frame "UI: Update Controls" {
            w438 = T3 {"Value"=10.0} ("Constant")
            # "Using Variant Attr. For Settings"
            n185 = Unbundle By Name(w453) -> ("Path Settings"=w452:refnum<class "Path Settings.lvclass">)
            n186 = property class="Path Settings.lvclass"(reference=w452) -> ("Accessors:Interpolation"=w451:dbl, "Accessors:Enabled"=w450:bool, "Accessors:Direction"=w449:u16, "Accessors:Fill Orientation"=w448:u16, "Accessors:Smooth Segments"=w446:dbl, "Accessors:Fill Spacing"=w445:dbl, "Accessors:Speed Schedule"=w447:u16, "Accessors:Voltage Schedule"=w444:u16, "Accessors:Resistance"=w443:T1, "Accessors:Deviate"=w433:bool, "Accessors:Speed Settings"=w437:variant, "Accessors:Voltage Settings"=w435:variant)  [unwired: 1 in, 2 out]
            n187 = local write "Interpolation"(w451) -> ()
            n188 = local write "Direction"(w449) -> ()
            n189 = local write "Smooth Segments"(w446) -> ()
            n190 = local write "Speed Schedule"(w447) -> ()
            n191 = local write "Set Resistance"(w443) -> ()
            n192 = call "Schedule.CheckVariantAttributes.vi"("Variant In"=w437) -> ("Variant Out"=w436:variant)  [unwired: 9 in, 1 out]
            n193 = call "Schedule.CheckVariantAttributes.vi"("Variant In"=w435) -> ("Variant Out"=w434:variant)  [unwired: 9 in, 1 out]
            n194 = local write "Enabled?"(w450) -> ()
            n195 = local write "Fill Orientation"(w448) -> ()
            n196 = local write "Fill Spacing"(w445) -> ()
            n197 = local write "Voltage Schedule"(w444) -> ()
            n198 = local write "Deviate?"(w433) -> ()
            n199 = call "Schedule.Read.vi"("Data to Read"=w438, "LUT In"=w436) -> ("Data Out"=w442:variant)  [unwired: 7 in, 2 out]
            n200 = call "Schedule.Read.vi"("Data to Read"=w438, "LUT In"=w434) -> ("Data Out"=w440:variant)  [unwired: 7 in, 2 out]
            n201 = Variant To Data(type=w438, Variant=w442) -> (data=w441:T3)  [unwired: 1 in, 1 out]
            n202 = Variant To Data(type=w438, Variant=w440) -> (data=w439:T3)  [unwired: 1 in, 1 out]
            n203 = Unbundle By Name(w441) -> ("Value"=w456:dbl)
            n204 = Unbundle By Name(w439) -> ("Value"=w455:dbl)
            n205 = local write "Speed (um/s)"(w456) -> ()
            n206 = local write "Voltage (V)"(w455) -> ()
            n207 = call <vilib>:"Add State(s) to Queue__jki_lib_state_machine.vi"("State(s) in (\"\")"=w459) -> ("States Out"=w458:string)  [unwired: 14 in]
          }
          frame "UI: Cursor Set" {
            # "Argument"
            # "Set and Unset Cursor Busy.\n(Usage: \"UI: Cursor Set >> Busy|Idle\")"
            n208 = case shown="\"Busy\"" w462 {
              tunnel: w464 -> [w468 w470]
              tunnel: [w467 w469] -> w463
              frame "Idle", Default {
                n209 = call <vilib>:"Unset Busy.vi"("error in (no error)"=w468) -> ("error out"=w467:errorcluster)  [unwired: 10 in]
              }
              frame "Busy" {
                n210 = call <vilib>:"Set Busy.vi"("error in (no error)"=w470) -> ("error out"=w469:errorcluster)  [unwired: 9 in, 1 out]
              }
            }
            n211 = call <vilib>:"Add State(s) to Queue__jki_lib_state_machine.vi"("State(s) in (\"\")"=w466) -> ("States Out"=w465:string)  [unwired: 14 in]
          }
          frame "UI: Update Speed/Voltage Visibility" {
            n212 = local read "Voltage Schedule"() -> (w479:u16)
            n213 = local read "Speed Schedule"() -> (w478:u16)
            n214 = case shown="1, Default" w479 {
              tunnel: [TRUE FALSE] -> w482
              frame 0 {
              }
              frame 1, Default {
              }
            }
            n215 = case shown="1, Default" w478 {
              tunnel: [TRUE FALSE] -> w480
              frame 0 {
              }
              frame 1, Default {
              }
            }
            n216 = property on="Voltage (V)" class="DigNum (strict)"(error in=w481, "Visible"=w482) -> (error out=w477:errorcluster)  [unwired: 1 in, 1 out]
            n217 = Not(x=w482) -> (.not. x?=w476:bool)
            n218 = property on="Voltage Settings" class="Bool (strict)"(error in=w477, "Visible"=w476) -> (error out=w475:errorcluster)  [unwired: 1 in, 1 out]
            n219 = property on="Speed (um/s)" class="DigNum (strict)"(error in=w475, "Visible"=w480) -> (error out=w474:errorcluster)  [unwired: 1 in, 1 out]
            n220 = Not(x=w480) -> (.not. x?=w472:bool)
            n221 = property on="Speed Settings" class="Bool (strict)"(error in=w474, "Visible"=w472) -> (error out=w473:errorcluster)  [unwired: 1 in, 1 out]
            n222 = call <vilib>:"Add State(s) to Queue__jki_lib_state_machine.vi"("State(s) in (\"\")"=w485) -> ("States Out"=w484:string)  [unwired: 14 in]
          }
          frame "UI: Front Panel State" {
            # "Argument"
            # "Set Front Panel Open or Closed\n(Usage: \"UI: Front Panel State >> Open|Close\")"
            n223 = Unbundle By Name(w490) -> ("Core.Current VI Reference"=w494:refnum<vi>)
            n224 = disable-structure shown="Default" {
              disable-tunnel: w492 -> [w501 w524]
              disable-tunnel: [w500 w524] -> w491
              disable-tunnel: w494 -> [w499 _]
              disable-tunnel: w493 -> [w498 _]
              frame condition #0 (active) {
                n225 = case shown="\"Close\"" w498 {
                  tunnel: w501 -> [w505 w518]
                  tunnel: [w507 w519] -> w500
                  tunnel: w499 -> [w506 w516]
                  frame "Open", Default {
                    n226 = property class="VI"(reference=w506, error in=w505) -> (reference out=w503:refnum<vi>, error out=w504:errorcluster, "FP.State"=w502:T8)
                    n227 = case shown="\"Closed\"" w502 {
                      tunnel: [w510 w513] -> w507
                      tunnel: w504 -> [w509 w513]
                      tunnel: w503 -> [w508 _]
                      frame "Closed" {
                        n228 = invoke class="VI" method="FP.Open"(reference=w508, error in=w509, "Activate"=TRUE, "State"=T8."Standard") -> (error out=w510:errorcluster)  [unwired: 1 in, 4 out]
                      }
                      frame Default {
                      }
                    }
                  }
                  frame "Close" {
                    n229 = property class="VI"(reference=w516, error in=w518) -> (reference out=w515:refnum<vi>, error out=w517:errorcluster, "FP.State"=w514:T8)
                    n230 = case shown="Default" w514 {
                      tunnel: [w520 w523] -> w519
                      tunnel: w517 -> [w520 w522]
                      tunnel: w515 -> [_ w521]
                      frame "Invalid", "Closed" {
                      }
                      frame Default {
                        n231 = invoke class="VI" method="FP.Close"(reference=w521, error in=w522) -> (error out=w523:errorcluster)  [unwired: 1 in, 2 out]
                      }
                    }
                  }
                }
              }
              frame condition #1 {
              }
            }
            n232 = call <vilib>:"Add State(s) to Queue__jki_lib_state_machine.vi"("State(s) in (\"\")"=w497) -> ("States Out"=w496:string)  [unwired: 14 in]
          }
          frame "---------- Process ----------" {
            # "Do not put any code in this frame.\n(It is a separator no-op. You can make a copy of this frame to create a new Macro frame)"
            n233 = call <vilib>:"Add State(s) to Queue__jki_lib_state_machine.vi"("State(s) in (\"\")"=w529) -> ("States Out"=w528:string)  [unwired: 14 in]
          }
          frame "Process: Sync" {
            # "Do not put any code in this frame.\n(It is a separator no-op. You can make a copy of this frame to create a new Macro frame)"
            n234 = Unbundle By Name(w533) -> ("Self"=w534:refnum<class "Edit.Path.lvclass">)
            n235 = call <vilib>:"WaitOnProcessSync.vi"("error in (no error)"=w531, "SMO"=w534) -> ("error out"=w532:errorcluster, "Don't run?"=w537:bool)  [unwired: 7 in, 1 out]
            n236 = Select(t="Data: Cleanup\nEvents: Unregister\nExit", s=w537, f="") -> (s? t:f=w530:string)
            n237 = call <vilib>:"Add State(s) to Queue__jki_lib_state_machine.vi"("State(s) in Front (\"\")"=w530, "State(s) in (\"\")"=w540) -> ("States Out"=w539:string)  [unwired: 13 in]
          }
          frame "---------- Macro ----------" {
            # "Do not put any code in this frame.\n(It is a separator no-op. You can make a copy of this frame to create a new Macro frame)"
            n238 = call <vilib>:"Add State(s) to Queue__jki_lib_state_machine.vi"("State(s) in (\"\")"=w545) -> ("States Out"=w544:string)  [unwired: 14 in]
          }
          frame "Macro: Initialize" {
            (unwired) "UI: Initialize\n//UI: Check Variants\n//UI: Update Controls\nUI: Update Speed/Voltage Visibility\nUI: Front Panel State >> Close"
            w547 = "Process: Sync"
            (unwired) "Data: Initialize\nInitialize Core Data\nDatabase: Locate\nEvents: Register\nUI: Initialize\n//UI: Check Variants\n//UI: Update Controls\nUI: Update Speed/Voltage Visibility\nUI: Front Panel State >> Close"
            # "Initialization Macro\n(This is called once, when the VI starts)"
            n239 = control-ref of="This VI"() -> (w549:refnum<vi>)
            n240 = property class="VI"(reference=w549) -> ("Exec.State"=w548:T9)  [unwired: 1 in, 2 out]
            n241 = Equal?(x=w548, y=T9."Run top level") -> (x = y?=w553:bool)
            n242 = Select(t=w547, s=w553, f="") -> ()  [unwired: 1 out]
            n243 = call <vilib>:"Add State(s) to Queue__jki_lib_state_machine.vi"("State(s) in Front (\"\")"="Data: Initialize\nInitialize Core Data\nDatabase: Locate\nEvents: Register", "State(s) in (\"\")"=w547, "State(s) at Back (\"\")"="UI: Initialize\n//UI: Check Variants\n//UI: Update Controls\nUI: Update Speed/Voltage Visibility\nUI: Front Panel State >> Close") -> ("States Out"=w546:string)  [unwired: 12 in]
            n244 = call <vilib>:"Add State(s) to Queue__jki_lib_state_machine.vi"("State(s) in Front (\"\")"=w546, "State(s) in (\"\")"=w559) -> ("States Out"=w558:string)  [unwired: 13 in]
          }
          frame "Macro: Exit" {
            # "Exit Macro\n(This is called once, when the VI exits)"
            n245 = Unbundle By Name(w570) -> ("Core.Close Panel on Exit?"=w561:bool)
            n246 = Select(t="UI: Front Panel State >> Close", s=w561, f="") -> (s? t:f=w566:string)
            n247 = call <vilib>:"Add State(s) to Queue__jki_lib_state_machine.vi"("State(s) in Front (\"\")"="Data: Cleanup\nEvents: Unregister", "State(s) in (\"\")"="Process: Sync", "State(s) at Back (\"\")"="Exit") -> ("States Out"=w563:string)  [unwired: 12 in]
            n248 = call <vilib>:"Add State(s) to Queue__jki_lib_state_machine.vi"("State(s) in (\"\")"=w566, "State(s) at Back (\"\")"=w563) -> ("States Out"=w560:string)  [unwired: 13 in]
            n249 = call <vilib>:"Add State(s) to Queue__jki_lib_state_machine.vi"("State(s) in Front (\"\")"=w560, "State(s) in (\"\")"=w573) -> ("States Out"=w572:string)  [unwired: 13 in]
          }
          frame "---------- Database ----------" {
            # "Template Separator\n(You can make a copy of, or modify, this frame)"
            n250 = call <vilib>:"Add State(s) to Queue__jki_lib_state_machine.vi"("State(s) in (\"\")"=w578) -> ("States Out"=w577:string)  [unwired: 14 in]
          }
          frame "Database: Copy to Group" {
            # "Template Separator\n(You can make a copy of, or modify, this frame)"
            n251 = Unbundle By Name(w587) -> ("SettingDB"=w586:refnum<class "Setting Database.lvclass">, "Path Settings"=w589:refnum<class "Path Settings.lvclass">)
            n252 = call-dynamic "Read Group.vi"("ObjectSettings in"=w589) -> ("Group"=w583:string)  [unwired: 8 in, 2 out]
            n253 = Bundle By Name(cluster=T10 {"Name"="", "Group"=""} ("Copy Settings To Group"), "Group"=w583, "Name"="p") -> (w581:T10)
            n254 = call "Setting Database.CopySettingsToGroup.vi"("error in (no error)"=w579, "Copy Settings To Group"=w581, "Setting Database"=w586) -> ("error out"=w580:errorcluster, "Setting Database out"=w584:refnum<class "Setting Database.lvclass">)  [unwired: 7 in]
            n255 = Bundle By Name(cluster=w587, "SettingDB"=w584) -> (w588:T14)
            n256 = call <vilib>:"Add State(s) to Queue__jki_lib_state_machine.vi"("State(s) in (\"\")"=w592) -> ("States Out"=w591:string)  [unwired: 14 in]
          }
          frame "Database: Set as Default" {
            # "Template Separator\n(You can make a copy of, or modify, this frame)"
            n257 = Unbundle By Name(w598) -> ("SettingDB"=w597:refnum<class "Setting Database.lvclass">)
            n258 = call "Setting Database.SetDefaultPath.vi"("error in (no error)"=w594, "SetDefaultPath"=T11 TRUE, "Setting Database"=w597) -> ("error out"=w595:errorcluster, "Setting Database out"=w596:refnum<class "Setting Database.lvclass">)  [unwired: 7 in]
            n259 = Bundle By Name(cluster=w598, "SettingDB"=w596) -> (w599:T14)
            n260 = call <vilib>:"Add State(s) to Queue__jki_lib_state_machine.vi"("State(s) in (\"\")"=w602) -> ("States Out"=w601:string)  [unwired: 14 in]
          }
          frame "Database: Locate" {
            # "#todo\nDecide what to do if not found..."
            # "Your code here.\n(You can make a copy of, or modify, this frame)"
            n261 = Unbundle By Name(w604) -> ("Self"=w610:refnum<class "Edit.Path.lvclass">, "SettingDB"=w613:refnum<class "Setting Database.lvclass">)
            n262 = call "Setting Database Name.vi"("error in (no error)"=w605) -> ("error out"=w606:errorcluster, "Name"=w603:string)  [unwired: 9 in]
            n263 = call <vilib>:"ListSharedResources.vi"("error in (no error)"=w606, "Filter (regex|name)"=w603, "SMO in"=w610) -> ("error out"=w607:errorcluster, "resources found?"=w611:bool, "Shared Resources"=w617:refnum<class "SMO.lvclass">[], "SMO out"=w609:refnum<class "Edit.Path.lvclass">)  [unwired: 5 in]
            n264 = case shown="True" w611 {
              tunnel: w617 -> [_ w630]
              tunnel: [w621 w626] -> w615
              tunnel: w613 -> [w621 w628]
              tunnel: w609 -> [w622 w627]
              tunnel: [w622 w627] -> w612
              tunnel: w607 -> [w620 w623]
              tunnel: [w620 w624] -> w608
              frame False {
              }
              frame True {
                n265 = Index Array(array=w630, index=0) -> (element=w629:refnum<class "SMO.lvclass">)
                n266 = To More Specific Class(target class=w628, reference=w629, error in=w623) -> (specific class reference=w626:refnum<class "Setting Database.lvclass">, error out=w624:errorcluster)
              }
            }
            n267 = Bundle By Name(cluster=w604, "Self"=w612, "SettingDB"=w615) -> (w616:T14)
            n268 = call <vilib>:"Add State(s) to Queue__jki_lib_state_machine.vi"("State(s) in (\"\")"=w619) -> ("States Out"=w618:string)  [unwired: 14 in]
          }
          frame "Database: Update Active" {
            # "Your code here.\n(You can make a copy of, or modify, this frame)"
            n269 = Unbundle By Name(w636) -> ("SettingDB"=w635:refnum<class "Setting Database.lvclass">, "Path Settings"=w633:refnum<class "Path Settings.lvclass">)
            n270 = call "Setting Database.UpdateActivePath.vi"("error in (no error)"=w631, "UpdateCurrentPath"=w633, "Setting Database"=w635) -> ("error out"=w632:errorcluster, "Setting Database"=w634:refnum<class "Setting Database.lvclass">)  [unwired: 7 in]
            n271 = Bundle By Name(cluster=w636, "SettingDB"=w634) -> (w637:T14)
            n272 = call <vilib>:"Add State(s) to Queue__jki_lib_state_machine.vi"("State(s) in (\"\")"=w640) -> ("States Out"=w639:string)  [unwired: 14 in]
          }
          frame "Database: Copy to All" {
            # "Template Separator\n(You can make a copy of, or modify, this frame)"
            n273 = Unbundle By Name(w646) -> ("SettingDB"=w645:refnum<class "Setting Database.lvclass">)
            n274 = call "Setting Database.CopyActivePathToAll.vi"("error in (no error)"=w641, "CopyActiveToAll"=T12 TRUE, "Setting Database"=w645) -> ("error out"=w642:errorcluster, "Setting Database out"=w644:refnum<class "Setting Database.lvclass">)  [unwired: 7 in]
            n275 = Bundle By Name(cluster=w646, "SettingDB"=w644) -> (w647:T14)
            n276 = call <vilib>:"Add State(s) to Queue__jki_lib_state_machine.vi"("State(s) in (\"\")"=w650) -> ("States Out"=w649:string)  [unwired: 14 in]
          }
        }
      }
    }
    frame Error {
    }
  }
  n277 = call-parent "Process.vi"("error in"=w7, "Edit"=w1) -> ("error out"=w5:errorcluster, "Edit out"=→"Edit.Path out":refnum<class "Edit.Path.lvclass">)  [unwired: 8 in]
  n278 = Merge Errors(w5, w4) -> (→"error out":errorcluster)
